vi "ximc fix usbser sys.vi"(8 "error in (no error)":errorcluster, 11 "device_uri":string) -> (0 "error out":errorcluster, 3 "function return":i32)   [LabVIEW 2012, in "libximc.lvlib"]
doc: "result_t XIMC_API ximc_fix_usbser_sys(const char* device_uri);"
uses:
  libximc.lvlib
  libximc.dll
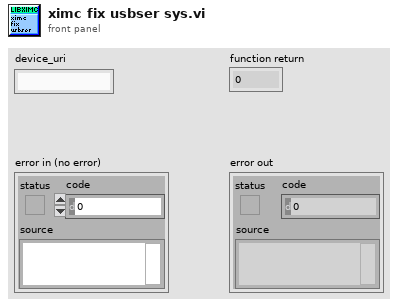
[diagram p1: front panel]
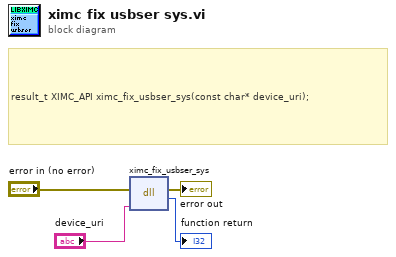
[diagram p0: block diagram]
diagram:
  # "result_t XIMC_API ximc_fix_usbser_sys(const char* device_uri);"
  n1 = dll-call lib="C:/Users/Vasily/Att_examples/LabVIEW_example/libximc.*" fn="ximc_fix_usbser_sys"(error in="error in (no error)", "device_uri"="device_uri") -> (error out=→"error out":errorcluster, →"function return":i32)  [unwired: 3 in, 1 out]
